vi "Execute.vi"(8 "error in":errorcluster, 11 "Change Filter Position in":refnum<class "Change Filter Position.lvclass">) -> (0 "error out":errorcluster, 1 "Next Step?":bool, 2 "MSG":string, 3 "Change Filter Position out":refnum<class "Change Filter Position.lvclass">)   [LabVIEW 2015, in "Change Filter Position.lvclass"]
uses:
  Change Filter Position.lvclass
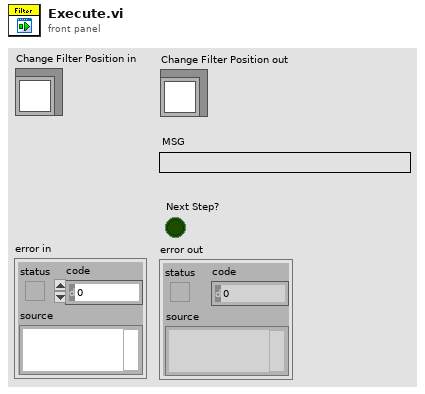
[diagram p1: front panel]
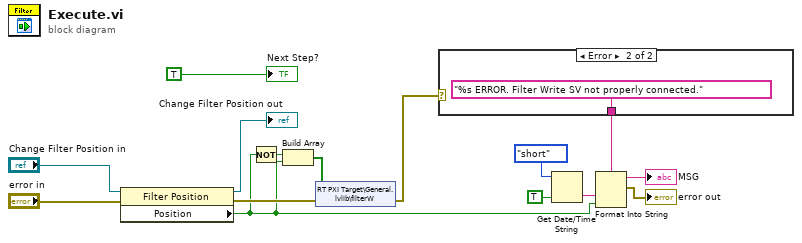
[diagram p0: block diagram]
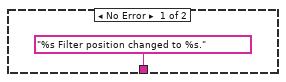
[diagram p2: hidden frame]
diagram:
  n1 = property class="Filter Position"(reference="Change Filter Position in", error in="error in") -> (reference out=→"Change Filter Position out":refnum<class "Change Filter Position.lvclass">, error out=w11:errorcluster, "Position"=w1:bool)
  n2 = Not(x=w1) -> (.not. x?=w2:bool)
  n3 = Build Array(w2, w1) -> (w4:bool[])
  n4 = shared-variable "RT PXI Target\\General.lvlib\\filterW"(w4, error in=w11) -> (error out=w3:errorcluster)
  n5 = case shown="Error" w3 {
    tunnel: ["%s Filter position changed to %s." ("format string") "%s ERROR. Filter Write SV not properly connected." ("format string")] -> w12
    frame No Error {
    }
    frame Error {
    }
  }
  n6 = Get Date/Time String(date format (0)=enum16{"short", "long", "abbreviated"}."short", want seconds? (F)=TRUE) -> (time string=w13:string)  [unwired: 1 in, 1 out]
  n7 = Format Into String(format string=w12, w13, w1) -> (resulting string=→"MSG":string, error out=→"error out":errorcluster)  [unwired: 2 in]
  "Next Step?" <- TRUE ("Next Step?")
